vi "AccelerometerAngularAccelerationCalculationLoop.vi"   [LabVIEW 2016]
uses:
  <vilib>/rvi/Emulation/niFpgaGetClockAttributes.vi
  <vilib>/rvi/Emulation/niFpgaSctlEmulationGetInTimedLoop.vi
  <vilib>/rvi/Emulation/niFpgaEmulationReportErrorSimple.vi
  <vilib>/rvi/Emulation/niFpgaEmulationIsFPGAContextNoSignature.vi
  <vilib>/rvi/errors/niFpgaSetErrorForExecOnDevCompSimple.vi
  <vilib>/rvi/eio/common/nirviEmuReportErrorAndStop.vi
  <vilib>/rvi/DataTransferAndStorage/Container/Common/niFpgaContainerGetUniqueNameForEmu.vi
  <vilib>/rvi/FIFO/Fifo_Resource/nirvififoEmulationSetSize.vi
  <vilib>/rvi/FIFO/Fifo_Resource/nirviFifoEmulationQueueMgr.vi
  <instcachedir>/0/nirviFifoEmulationQueueMgr_E5CAEC123FF24DC58D834DCA3CDAA9B5.lvgen/nirviFifoEmulationQueueMgr_E5CAEC123FF24DC58D834DCA3CDAA9B5_026.vi
  <vilib>/Utility/error.llb/Clear Errors.vi
  <vilib>/rvi/FIFO/Fifo_Resource/nirvififoEmulationCreateLock.vi
  <vilib>/rvi/Emulation/niFpgaProcessEmulError.vi
  <vilib>/rvi/FIFO/Fifo_Resource/nirvififoEmulationObtainLock.vi
  <vilib>/rvi/FIFO/Fifo_Resource/nirvififoEmulationReleaseLock.vi
  <vilib>/rvi/occurrence/nirviWaitOnOccurrenceBase.vi
  <vilib>/rvi/errors/nirviReportUnexpectedCaseInternalError.vi
  <vilib>/rvi/errors/nirviReportUnexpectedCaseInternalError (U32).vi
  <userlib>/_NI FLP Library/FPGA/outsideSCTL/FlpLib Add Shared Instance 0.vi
  <userlib>/_NI FLP Library/FPGA/outsideSCTL/FlpLib Subtract Shared Instance 0.vi
  <userlib>/_NI FLP Library/FPGA/outsideSCTL/FlpLib Divide Shared Instance 0.vi
  <vilib>/rvi/FIFO/Fifo_Resource/nirvififoEmulationDetermineInputValidOut.vi
  <vilib>/rvi/Emulation/niFpgaCriticalErrorInLSC.vi
  <vilib>/rvi/DataTransferAndStorage/Container/XNode/niFpgaContainer.xnode
  <vilib>/rvi/FIFO/Fifo_Resource/nirvififoEmulationRead.vi
  <vilib>/rvi/FIFO/Fifo_Resource/nirvififoEmulationWrite.vi
types:
  T1 = cluster{"Timestamp":u64, "Accelerometer1Voltage":sgl, "Accelerometer2Voltage":sgl, "Accelerometer3Voltage":sgl, "Accelerometer4Voltage":sgl, "Accelerometer5Voltage":sgl, "Accelerometer6Voltage":sgl, "Accelerometer7Voltage":sgl, "Accelerometer8Voltage":sgl, "Accelerometer1Acceleration":sgl, "Accelerometer2Acceleration":sgl, "Accelerometer3Acceleration":sgl, "Accelerometer4Acceleration":sgl, "Accelerometer5Acceleration":sgl, "Accelerometer6Acceleration":sgl, "Accelerometer7Acceleration":sgl, "Accelerometer8Acceleration":sgl, "AngularAccelerationX":sgl, "AngularAccelerationY":sgl, "AngularAccelerationZ":sgl}
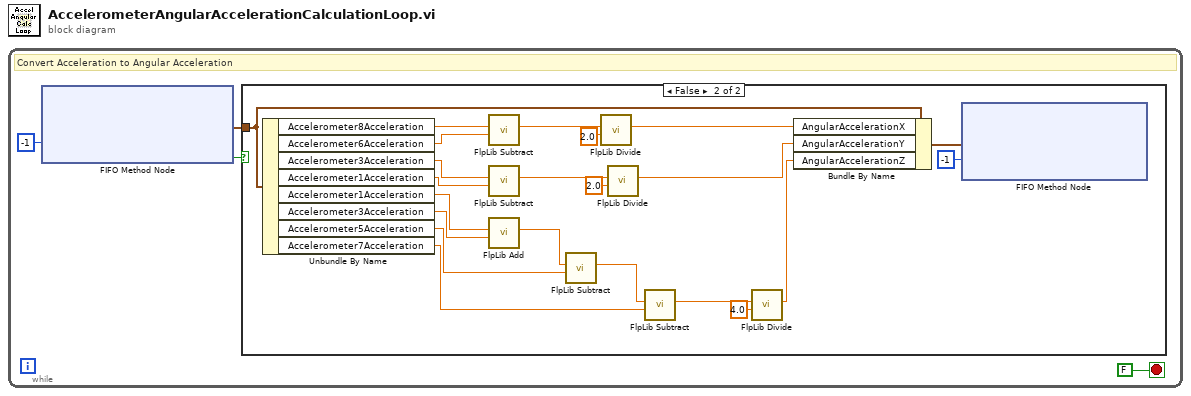
[diagram p0: block diagram]
diagram:
  n1 = while {
    stop <- FALSE stop-if-true
    # "Convert Acceleration to Angular Acceleration"
    n2 = xnode ("FIFO Method Node")("Timeout"=-1) -> ("Element"=w2:T1, "Timed Out?"=w3:bool)  [unwired: 1 in, 1 out]
    n3 = case shown="False" w3 {
      tunnel: w2 -> [_ w18]
      frame True {
      }
      frame False {
        n4 = Unbundle By Name(w18) -> ("Accelerometer8Acceleration"=w17:sgl, "Accelerometer6Acceleration"=w16:sgl, "Accelerometer3Acceleration"=w14:sgl, "Accelerometer1Acceleration"=w13:sgl, "Accelerometer1Acceleration"=w12:sgl, "Accelerometer3Acceleration"=w11:sgl, "Accelerometer5Acceleration"=w10:sgl, "Accelerometer7Acceleration"=w9:sgl)
        n5 = call-poly <userlib>:"FlpLib Subtract.vi"("y"=w16, "x"=w17) -> ("x-y"=w26:sgl)  [unwired: 5 in]
        n6 = call-poly <userlib>:"FlpLib Subtract.vi"("y"=w13, "x"=w14) -> ("x-y"=w23:sgl)  [unwired: 5 in]
        n7 = call-poly <userlib>:"FlpLib Add.vi"("y"=w11, "x"=w12) -> ("x+y"=w22:sgl)  [unwired: 5 in]
        n8 = call-poly <userlib>:"FlpLib Subtract.vi"("y"=w10, "x"=w22) -> ("x-y"=w21:sgl)  [unwired: 5 in]
        n9 = call-poly <userlib>:"FlpLib Divide.vi"("y"=sgl 2.0, "x"=w26) -> ("x/y"=w15:sgl)  [unwired: 5 in]
        n10 = call-poly <userlib>:"FlpLib Divide.vi"("y"=sgl 2.0, "x"=w23) -> ("x/y"=w8:sgl)  [unwired: 5 in]
        n11 = call-poly <userlib>:"FlpLib Subtract.vi"("y"=w9, "x"=w21) -> ("x-y"=w19:sgl)  [unwired: 5 in]
        n12 = call-poly <userlib>:"FlpLib Divide.vi"("y"=sgl 4.0, "x"=w19) -> ("x/y"=w7:sgl)  [unwired: 5 in]
        n13 = Bundle By Name(cluster=w18, "AngularAccelerationX"=w15, "AngularAccelerationY"=w8, "AngularAccelerationZ"=w7) -> (w5:T1)
        n14 = xnode ("FIFO Method Node")("Element"=w5, "Timeout"=-1) -> ()  [unwired: 1 in, 2 out]
      }
    }
  }
